vi "FPGA Main Default.vi"() -> ()   [LabVIEW 2019]
doc: "The myRIO v1.1 FPGA Shipping Personality. This personality contains support for:\n- 2 Analog Input Interrupt channel\n- 4 Digital Input Interrupt channel\n- 1 Timer\n- 1 Accelerometer\n- 1 Button\n- 4 LED\n- 10 Analog Input channels with 1 Sample\n- 6 Analog Output channels with 1 Sample\n- 40 Digital I/O channels with 1 Sample\n- 2 I2C channels\n- 4 Encoder channels\n- 6 PWM channels\n- 2 SPI channels"
uses:
  Sub VIs/Utilities/Start Boolean.ctl
  <vilib>/Platform/TimedLoop/XDataNode/timing_clust.ctl
  <vilib>/Platform/TimedLoop/XDataNode/nitl_modes.ctl
  <vilib>/Platform/TimedLoop/XDataNode/wakeup.ctl
  <vilib>/rvi/Emulation/niFpgaGetClockAttributes.vi
  <vilib>/rvi/Emulation/niFpgaSctlEmulationGetInTimedLoop.vi
  <vilib>/rvi/Emulation/niFpgaEmulationReportErrorSimple.vi
  <vilib>/rvi/eio/common/nirviEmuTemplateMethod_errors.vi
  <vilib>/rvi/Emulation/niFpgaCriticalErrorInLSC.vi
  <vilib>/rvi/Emulation/niFpgaProcessEmulError.vi
  <vilib>/rvi/Emulation/niFpgaEmulationIsFPGAContextNoSignature.vi
  <vilib>/rvi/errors/niFpgaSetErrorForExecOnDevCompSimple.vi
  <vilib>/rvi/eio/common/nirviEmuReportErrorAndStop.vi
  <vilib>/rvi/DataTransferAndStorage/Container/Common/niFpgaContainerGetUniqueNameForEmu.vi
  <vilib>/rvi/FIFO/Fifo_Resource/nirvififoEmulationSetSize.vi
  <vilib>/rvi/FIFO/Fifo_Resource/nirviFifoEmulationQueueMgr.vi
  <instcachedir>/0/nirviFifoEmulationQueueMgr_E5CAEC123FF24DC58D834DCA3CDAA9B5.lvgen/nirviFifoEmulationQueueMgr_E5CAEC123FF24DC58D834DCA3CDAA9B5_000.vi
  <vilib>/rvi/FIFO/Fifo_Resource/nirvififoEmulationDetermineInputValidOut.vi
  <vilib>/rvi/FIFO/Fifo_Resource/nirvififoEmulationCreateLock.vi
  <vilib>/rvi/FIFO/Fifo_Resource/nirvififoEmulationObtainLock.vi
  <vilib>/rvi/FIFO/Fifo_Resource/nirvififoEmulationReleaseLock.vi
  <vilib>/rvi/occurrence/nirviWaitOnOccurrenceBase.vi
  <vilib>/rvi/errors/nirviReportUnexpectedCaseInternalError.vi
  <vilib>/rvi/errors/nirviReportUnexpectedCaseInternalError (U32).vi
  <vilib>/Utility/error.llb/Clear Errors.vi
  <vilib>/rvi/DataTransferAndStorage/Container/Common/niFpgaContainerExecOnDevCompGetState.vi
  <instcachedir>/0/nirviFifoEmulationQueueMgr_E5CAEC123FF24DC58D834DCA3CDAA9B5.lvgen/nirviFifoEmulationQueueMgr_E5CAEC123FF24DC58D834DCA3CDAA9B5_001.vi
  <vilib>/rvi/interface/RandomDataEmulation/niFpgaRandomDataHandleErrors.vi
  <vilib>/rvi/DataTransferAndStorage/Container/Common/niFpgaContainerSetEmuInfo.vi
  <vilib>/eio/EIONode/EIONode.xnode
  <vilib>/rvi/DataTransferAndStorage/Container/XNode/niFpgaContainer.xnode
  <vilib>/rvi/FIFO/Fifo_Resource/nirvififoEmulationWrite.vi
  <vilib>/rvi/FIFO/Fifo_Resource/nirvififoEmulationRead.vi
  <vilib>/Platform/TimedLoop/XDataNode/XDataNode.xnode
  <vilib>/rvi/FIFO/Fifo_Resource/niFpgaFifoEmulationRefIn.vi
  <vilib>/rvi/LocalResourceManager/LocalResourceManager.xnode
  <vilib>/Platform/TimedLoop/XDataNode/XDNodeRunTimeDep.lvlib
panel:
  in  "AO.A_0.VAL":u16
  in  "AO.A_1.VAL":u16
  in  "AO.B_0.VAL":u16
  in  "AO.B_1.VAL":u16
  out "AI.B_3.VAL":u16
  out "AI.B_2.VAL":u16
  out "AI.B_1.VAL":u16
  out "AI.B_0.VAL":u16
  out "AI.A_3.VAL":u16
  out "AI.A_2.VAL":u16
  out "AI.A_1.VAL":u16
  out "AI.A_0.VAL":u16
  in  "PWM.A_2.CS":u8=1
  in  "PWM.A_2.CNFG":u8=4
  out "PWM.A_2.CNTR":u16
  in  "PWM.A_2.MAX":u16=39999
  in  "PWM.A_2.CMP":u16=20000
  in  "PWM.A_1.CS":u8=1
  in  "PWM.A_1.CNFG":u8=4
  out "PWM.A_1.CNTR":u16
  in  "PWM.A_1.MAX":u16=39999
  in  "PWM.A_1.CMP":u16=20000
  in  "PWM.A_0.CS":u8=1
  in  "PWM.A_0.CNFG":u8=4
  out "PWM.A_0.CNTR":u16
  in  "PWM.A_0.CMP":u16=20000
  in  "PWM.A_0.MAX":u16=39999
  in  "SPI.A.DATO":u16
  out "SPI.A.DATI":u16
  in  "SPI.A.CNFG":u16=112
  in  "SPI.A.CNT":u16=19
  in  "ENC.A.CNFG":u8 format="%08b"
  out "ENC.A.CNTR":u32
  out "ENC.A.STAT":u8 format="%08b"
  in  "SPI.A.GO":T1
  out "SPI.A.STAT":u8 format="%08b"
  out "I2C.A.STAT":u8 format="%08b"
  in  "I2C.A.CNTL":u8 format="%08b"
  in  "I2C.A.CNTR":u8=213
  in  "I2C.A.ADDR":u8 format="%08b"
  out "I2C.A.DATI":u8
  in  "I2C.A.DATO":u8
  in  "I2C.A.CNFG":u8=1 format="%08b"
  in  "I2C.A.GO":T1
  out "SYS.AI.RDY":bool
  out "SYS.RDY":bool
  out "DIO.A_7:0.IN":u8 format="%08b"
  in  "DIO.A_7:0.OUT":u8 format="%08b"
  in  "DIO.A_7:0.DIR":u8 format="%08b"
  out "DIO.C_7:0.IN":u8 format="%08b"
  in  "DIO.C_7:0.DIR":u8 format="%08b"
  in  "DIO.C_7:0.OUT":u8 format="%08b"
  out "AI.C_1.VAL":u16
  out "AI.C_0.VAL":u16
  in  "AO.C_0.VAL":u16
  in  "AO.C_1.VAL":u16
  in  "SYS.SELECTC":u8 format="%08b"
  in  "SYS.SELECTA":u8 format="%08b"
  in  "ENC.C_0.CNFG":u8 format="%08b"
  out "ENC.C_0.CNTR":u32
  out "ENC.C_0.STAT":u8 format="%08b"
  in  "ENC.C_1.CNFG":u8 format="%08b"
  out "ENC.C_1.CNTR":u32
  out "ENC.C_1.STAT":u8 format="%08b"
  in  "PWM.C_1.CS":u8=1
  in  "PWM.C_1.CNFG":u8=4
  out "PWM.C_1.CNTR":u16
  in  "PWM.C_1.CMP":u16=20000
  in  "PWM.C_1.MAX":u16=39999
  in  "PWM.C_0.CS":u8=1
  in  "PWM.C_0.CNFG":u8=4
  out "PWM.C_0.CNTR":u16
  in  "PWM.C_0.CMP":u16=20000
  in  "PWM.C_0.MAX":u16=39999
  out "DIO.A_15:8.IN":u8 format="%08b"
  in  "DIO.A_15:8.OUT":u8 format="%08b"
  in  "DIO.A_15:8.DIR":u8 format="%08b"
  out "AI.AudioIn_R.VAL":u16
  out "AI.AudioIn_L.VAL":u16
  in  "AO.AudioOut_R.VAL":u16
  in  "AO.AudioOut_L.VAL":u16
  in  "AO.SYS.GO":T1
  out "ACC.X.VAL":u16
  out "ACC.Y.VAL":u16
  out "SYS.ACC.RDY":bool
  out "ACC.Z.VAL":u16
  in  "DO.LED3:0":u8 format="%04b"
  out "DI.BTN":u8 format="%08b"
  out "AO.SYS.STAT":bool
  in  "IRQ.AI_A_3:0.CNFG":u8 format="%.0b"
  in  "IRQ.AI_A_0.THRESHOLD":u16
  in  "IRQ.AI_A_1.THRESHOLD":u16
  in  "IRQ.AI_A_0.NO":u8
  in  "IRQ.AI_A_1.NO":u8
  in  "IRQ.DIO_A_7:0.ENA":u8 format="%08b"
  in  "IRQ.DIO_A_7:0.RISE":u8 format="%08b"
  in  "IRQ.DIO_A_7:0.FALL":u8 format="%08b"
  in  "IRQ.DIO_A_0.NO":u8
  in  "IRQ.DIO_A_1.NO":u8
  in  "IRQ.DIO_A_2.NO":u8
  in  "IRQ.DIO_A_3.NO":u8
  in  "IRQ.DIO_A_3.CNT":u32
  in  "IRQ.DIO_A_2.CNT":u32
  in  "IRQ.DIO_A_1.CNT":u32
  in  "IRQ.DIO_A_0.CNT":u32
  in  "IRQ.AI_A_1.HYSTERESIS":u16=17
  in  "IRQ.TIMER.WRITE":u32
  in  "IRQ.TIMER.SETTIME":T1
  out "IRQ.TIMER.READ":u32
  in  "SPI.A.IRQ.NO":u8=15
  in  "IRQ.AI_A_0.HYSTERESIS":u16=17
  in  "IRQ.DI_BTN.ENA":bool
  in  "IRQ.DI_BTN.RISE":bool
  in  "IRQ.DI_BTN.FALL":bool
  in  "IRQ.DI_BTN.CNT":u32
  in  "IRQ.DI_BTN.NO":u8
  # "System"
  # "Onboard Devices"
  # "Connector A"
  # "Connector B"
  # "Connector C"
  # "Audio Connector"
  # "Accelerometer"
  # "Analog Input"
  # "Analog Output"
  # "Digital I/O"
  # "PWM"
  # "SPI Master"
  # "Analog Input"
  # "Analog Output"
  # "Digital I/O"
  # "PWM"
  # "SPI Master"
  # "Analog Input"
  # "Analog Output"
  # "Digital I/O"
  # "Counters / PWM"
  # "Analog Input"
  # "Analog Output"
  # "IO Configuration"
  # "IO Configuration"
  # "IO Configuration"
  # "Encoders"
  # "Buttons & LEDs"
  # "Analog Interrupt"
  # "Digital Interrupt"
  # "Encoders"
  # "Encoders"
  # "Button Interrupt"
  # "I2C Master"
  # "I2C Master"
  # "Timer Interrupt"
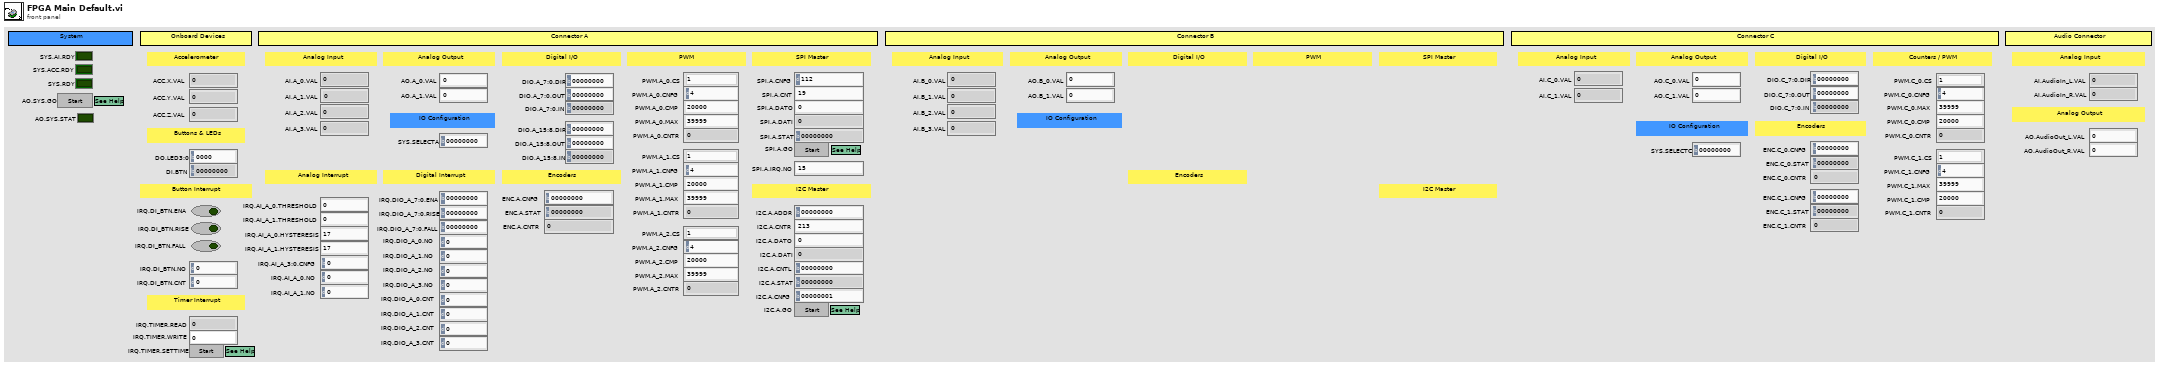
[diagram p1: front panel]
types:
  T1 = typedef "Start Boolean.ctl" = bool
  T2 = typedef "XDNodeRunTimeDep.lvlib/timing_clust.ctl" = cluster{"Expected End [f-1]":u64, "Actual End [f-1]":u64, "Finished Late? [f-1]":bool, "Expected End [i-1]":u64, "Actual End [i-1]":u64, "Finished Late? [i-1]":bool, "Expected Start [i]":u64, "Actual Start [i]":u64, "Expected Start [f]":u64, "Actual Start [f]":u64, "Source Name":string, "Structure Name":string, "Period":i64, "Deadline":i64, "Offset":i64, "Start":i64, "Priority":i32, "Timeout":i32, "Mode":T3, "Wakeup Reason":T4, "Error":errorcluster, "Source Type":string, "Secondary Source Type":string, "Global End Time":u64, "Global Start Time":u64, "Frame Duration":u64, "Iteration Duration":u64, "Assigned CPU":i32, "I/O Scan Engine Mode":u32}
  T3 = typedef "XDNodeRunTimeDep.lvlib/nitl_modes.ctl" = enum32{"No Change", "Process missed periods, maintain original phase", "Discard missed periods, maintain original phase", "Process missed periods, ignore original phase", "Discard missed periods, ignore original phase"}
  T4 = typedef "XDNodeRunTimeDep.lvlib/wakeup.ctl" = enum32{"Normal", "Aborted", "Asynchronous wakeup", "Timing source error", "Timed loop error", "Timeout"}
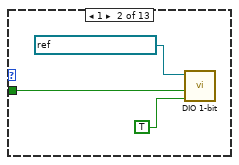
[diagram p3: hidden frame]
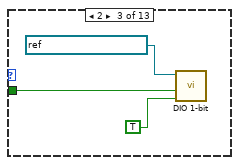
[diagram p4: hidden frame]
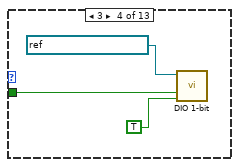
[diagram p5: hidden frame]
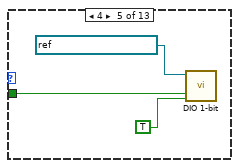
[diagram p6: hidden frame]
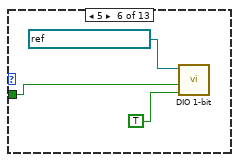
[diagram p7: hidden frame]
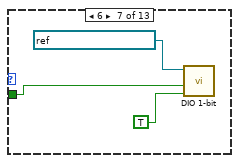
[diagram p8: hidden frame]
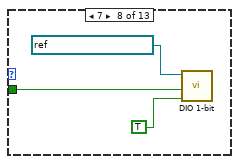
[diagram p9: hidden frame]
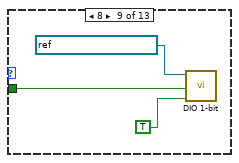
[diagram p10: hidden frame]
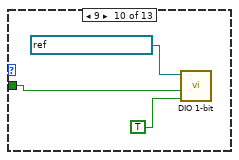
[diagram p11: hidden frame]
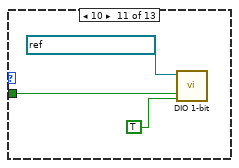
[diagram p12: hidden frame]
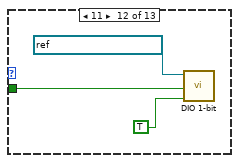
[diagram p13: hidden frame]
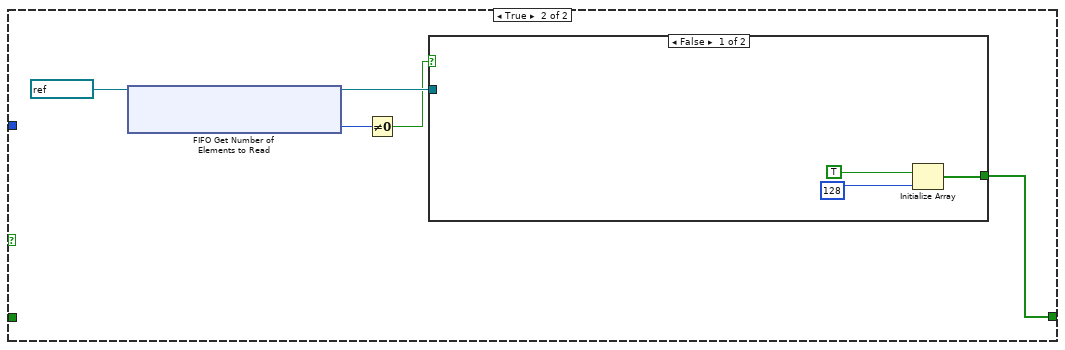
[diagram p15: hidden frame]
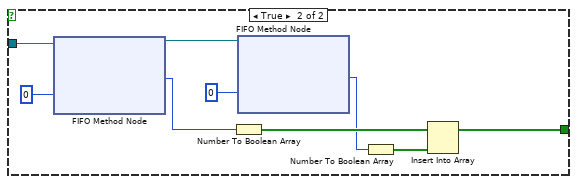
[diagram p16: hidden frame]
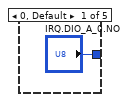
[diagram p19: hidden frame]
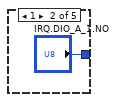
[diagram p20: hidden frame]
diagram:
  # "The Timed Loop does not allow writing the same FIFO outside the Timed Loop. Use another FIFO to push all interrupts from Button in the Timed Loop to the IRQ Queue."
  # "The Timed Loop does not allow writing the same FIFO outside the Timed Loop. Use another FIFO to push all interrupts from DIO in the Timed Loop to the IRQ Queue."
  # "The accelerometer nodes take some time before the FPGA can first read the values. This is because it takes time to read from the accelerometer. An iteration of the While Loop will not complete until the accelerometer values have been read.\n\nAfter the completion of the first iteration of the While Loop, all indicators have valid values."
  # "The analog output nodes take some time before the FPGA write the values to the pins. The GO and STAT registers are used to handshake between the FPGA and host. When the host wants the values to be written, the host sets the GO register to TRUE. If the host reads the STAT register before setting the value of the GO register, it can wait for the value of the STAT register to invert. The value inversion tells the host that the output values have been written."
  # "The analog input nodes take some time before the FPGA can first read the values. This is because it takes time to set up the Analog-to-Digital converter (ADC) and convert the first reading. An iteration of the While Loop will not complete until all the analog input channels have been sampled.\n\nAfter the completion of the first iteration of the While Loop, all indicators have valid values."
  # "Note: On some hardware a \"ghosting effect\" may occur on any unconnected AI channels. For example, if channel AI0 is connected and channels AI1~AI7 are not connected the the value read at AI0 may be seen on indicators AI1~AI7. This is common for hardware that use a multiplexed (MUXed) Analog-to-Digital converter (ADC), because the input analog signal is used to charge a capacitor which does not discharge before the unconnected channel is read.\n\nYou can hide the \"ghosting effect\" by using an mask register. This register is used to decide when the indicator should be updated."
  # "The FPGA timer fires the interrupt request (IRQ) when TIMER.Read counts down to zero. If TIMER.Read is not zero, it counts down to one per microsecond."
  # "The only interface that sends interrupts to the RT side. Timer interrupts, analog input interrupts, digital input interrupts, and SPI interrupt share this interface.\n\nAll interrupts work in sequence. One interrupt waits until the previous interrupt request (IRQ) gets acknowledged on the RT side."
  # "NOTE: The SYS.RDY Boolean MUST exist and must become TRUE at some point. Otherwise, the myRIO VIs will not function correctly."
  # "There is some delay between the time when the FPGA code starts and the time when the analog inputs, accelerometer, and scaling values outputs are valid. If the host wants to ensure that there are valid values in theses registers it should wait for each subsystem to finish its initialization process. \n\nWhen all subsystems have finished initializinig, the SYS.RDY indicator turns true. The host can poll the SYS.RDY indicator to determine the status of the FPGA. Alternatively, the host can poll the individual SYS.xx.RDY indicators to determine the status of the individual subsystems.\n\nThis loop continues indefinitely, essentially making SYS.RDY a read-only register."
  n1 = while {
    stop <- FALSE stop-if-true
    # "Host Synchronization"
    n2 = local read "SYS.ACC.RDY"() -> (w13:bool)
    n3 = local read "SYS.AI.RDY"() -> (w15:bool)
    n4 = Compound Arithmetic op=AND(w15, w13) -> (→"SYS.RDY":bool)
  }
  n5 = while {
    stop <- FALSE stop-if-true
    # "Interrupt to RT"
    n6 = xnode ("FIFO Method Node")("Timeout"=-1) -> ("Element"=w18:u8)  [unwired: 1 in, 2 out]
    n7 = call <vilib>:"niFPGA Interrupt.vi"("Wait Until Cleared (F)"=TRUE, "IRQ Number (0)"=w18) -> ()  [unwired: 1 in]
  }
  n8 = while {
    stop <- FALSE stop-if-true
    # "Timer"
    n9 = local read "IRQ.TIMER.READ"() -> (w23:u32)
    n10 = Select(t="IRQ.TIMER.WRITE", s="IRQ.TIMER.SETTIME", f=w23) -> (s? t:f=w21:u32)
    n11 = case shown="Default" w21 {
      selector: w21 -> [w27 w30]
      tunnel: [w27 w28] -> w20
      frame 0 {
      }
      frame Default {
        n12 = Decrement(x=w30) -> (x-1=w29:u32)
        n13 = case shown="0" w29 {
          selector: w29 -> [w31 w34]
          tunnel: [w31 w34] -> w28
          frame Default {
          }
          frame 0 {
            w33 = u8 0  # Reserved for Timer IRQ
            n14 = xnode ("FIFO Method Node")("Element"=w33, "Timeout"=-1) -> ()  [unwired: 1 in, 2 out]
          }
        }
      }
    }
    "IRQ.TIMER.READ" <- w20
    n15 = call "Loop Timer"("Count(uSec)"=u8 1 ("Count(mSec)")) -> ()  [unwired: 1 out]
  }
  n16 = xnode "VI-Defined FIFO Configuration"() -> ("FIFO Out"=w3:refnum<k21>)
  n17 = while {
    tunnel: w3 -> [w36]
    i -> [w63]
    stop <- FALSE stop-if-true
    # "Analog Input"
    n18 = xnode "FPGA I/O Node"() -> ("ConnectorA/AI0"=w41:u16, "ConnectorA/AI1"=w40:u16, "ConnectorA/AI2"=→"AI.A_2.VAL":u16, "ConnectorA/AI3"=→"AI.A_3.VAL":u16, "ConnectorB/AI0"=→"AI.B_0.VAL":u16, "ConnectorB/AI1"=→"AI.B_1.VAL":u16, "ConnectorB/AI2"=→"AI.B_2.VAL":u16, "ConnectorB/AI3"=→"AI.B_3.VAL":u16, "ConnectorC/AI0"=w57:i16, "ConnectorC/AI1"=w56:i16, "AudioIn/Left"=w55:i16, "AudioIn/Right"=w54:i16)  [unwired: 12 in, 12 out]
    "AI.A_0.VAL" <- w41
    "AI.A_1.VAL" <- w40
    n19 = Greater Than 0?(x=w63) -> (x > 0?=→"SYS.AI.RDY":bool)
    n20 = Number To Boolean Array(number="IRQ.AI_A_3:0.CNFG") -> (Boolean array=w51:bool[])
    n21 = Index Array(array=w51) -> (element #1=w49:bool, element #2=w48:bool, element #3=w46:bool, element #4=w45:bool)  [unwired: 4 in]
    n22 = To Unsigned Word Integer(number=w57) -> (unsigned 16bit integer=→"AI.C_0.VAL":u16)
    n23 = To Unsigned Word Integer(number=w56) -> (unsigned 16bit integer=→"AI.C_1.VAL":u16)
    n24 = To Unsigned Word Integer(number=w55) -> (unsigned 16bit integer=→"AI.AudioIn_L.VAL":u16)
    n25 = To Unsigned Word Integer(number=w54) -> (unsigned 16bit integer=→"AI.AudioIn_R.VAL":u16)
    n26 = call "Check AI IRQ.vi"("Hysteresis"="IRQ.AI_A_1.HYSTERESIS", "FIFO In"=w36, "IRQ Number"="IRQ.AI_A_1.NO", "Threshold"="IRQ.AI_A_1.THRESHOLD", "Analog Value"=w40, "Rising Edge?"=w45, "Enable Interrupt?"=w46) -> ()  [unwired: 5 in]
    n27 = call "Check AI IRQ.vi"("Hysteresis"="IRQ.AI_A_0.HYSTERESIS", "FIFO In"=w36, "IRQ Number"="IRQ.AI_A_0.NO", "Threshold"="IRQ.AI_A_0.THRESHOLD", "Analog Value"=w41, "Rising Edge?"=w48, "Enable Interrupt?"=w49) -> ()  [unwired: 5 in]
  }
  n28 = while {
    stop <- FALSE stop-if-true
    # "Analog Output"
    n29 = feedback #1(FALSE) -> (w69:bool)
    n30 = case shown="True" "AO.SYS.GO" {
      tunnel: "AO.C_0.VAL" -> [_ w91]
      tunnel: "AO.C_1.VAL" -> [_ w90]
      tunnel: "AO.A_0.VAL" -> [_ w95]
      tunnel: "AO.A_1.VAL" -> [_ w94]
      tunnel: "AO.B_0.VAL" -> [_ w93]
      tunnel: "AO.B_1.VAL" -> [_ w92]
      tunnel: "AO.AudioOut_L.VAL" -> [_ w87]
      tunnel: "AO.AudioOut_R.VAL" -> [_ w86]
      tunnel: w69 -> [w80 w83]
      tunnel: [w80 w81] -> w67
      frame False {
      }
      frame True {
        n31 = To Word Integer(number=w91) -> (16bit integer=w89:i16)
        n32 = To Word Integer(number=w90) -> (16bit integer=w88:i16)
        n33 = To Word Integer(number=w87) -> (16bit integer=w85:i16)
        n34 = To Word Integer(number=w86) -> (16bit integer=w84:i16)
        n35 = flat-sequence {
          tunnel: w95 -> [w104]
          tunnel: w94 -> [w103]
          tunnel: w93 -> [w102]
          tunnel: w92 -> [w101]
          tunnel: w89 -> [w100]
          tunnel: w88 -> [w99]
          tunnel: w85 -> [w98]
          tunnel: w84 -> [w97]
          tunnel: w83 -> [w96]
          tunnel: [w96] -> w82
          tunnel: w82 -> [w106]
          tunnel: [w105] -> w81
          frame #0 {
            n36 = xnode "FPGA I/O Node"("ConnectorA/AO0"=w104, "ConnectorA/AO1"=w103, "ConnectorB/AO0"=w102, "ConnectorB/AO1"=w101, "ConnectorC/AO0"=w100, "ConnectorC/AO1"=w99, "AudioOut/Left"=w98, "AudioOut/Right"=w97) -> ()  [unwired: 8 in, 8 out]
          }
          frame #1 {
            n37 = Not(x=w106) -> (.not. x?=w105:bool)
          }
        }
      }
    }
    "AO.SYS.STAT" <- w67
    n38 = feedback-in #1(w67) -> ()
  }
  n39 = while {
    i -> [w111]
    stop <- FALSE stop-if-true
    # "Onboard Accelerometer"
    n40 = xnode "FPGA I/O Node"() -> ("AccelerationX"=w114:i16, "AccelerationY"=w113:i16, "AccelerationZ"=w112:i16)  [unwired: 3 in, 3 out]
    n41 = Greater Than 0?(x=w111) -> (x > 0?=→"SYS.ACC.RDY":bool)
    n42 = To Unsigned Word Integer(number=w114) -> (unsigned 16bit integer=→"ACC.X.VAL":u16)
    n43 = To Unsigned Word Integer(number=w113) -> (unsigned 16bit integer=→"ACC.Y.VAL":u16)
    n44 = To Unsigned Word Integer(number=w112) -> (unsigned 16bit integer=→"ACC.Z.VAL":u16)
  }
  n45 = xnode "VI-Defined FIFO Configuration"() -> ("FIFO Out"=w2:refnum<k21>)
  n46 = node-c288() -> (w5:T2)  [unwired: 1 in]
  n47 = timed-loop {
    timing: w5 -> [_]
    timing-out: [_] -> w4
    tunnel: w2 -> [w118]
    stop <- _ stop-if-true
    # "Onboard DIO"
    n48 = xnode "FPGA I/O Node"() -> ("Button0"=w122:bool)  [unwired: 1 in, 1 out]
    n49 = Number To Boolean Array(number="DO.LED3:0") -> (Boolean array=w127:bool[])
    n50 = Build Array(w122) -> (w130:bool[])
    n51 = Index Array(array=w127) -> (element #1=w126:bool, element #2=w125:bool, element #3=w124:bool, element #4=w123:bool)  [unwired: 4 in]
    n52 = call "DIO IRQ 1-bit.vi"("IRQ.NO"="IRQ.DI_BTN.NO", "IRQ.CNT"="IRQ.DI_BTN.CNT", "FIFO in"=w118, "IRQ.FALL"="IRQ.DI_BTN.FALL", "IRQ.RISE"="IRQ.DI_BTN.RISE", "IRQ.ENA"="IRQ.DI_BTN.ENA", "DIO"=w122) -> ()  [unwired: 5 in]
    n53 = Boolean Array To Number(Boolean array=w130) -> (number=→"DI.BTN":u8)
    n54 = xnode "FPGA I/O Node"("LED0"=w126, "LED1"=w125, "LED2"=w124, "LED3"=w123) -> ()  [unwired: 4 in, 4 out]
  }
  n55 = while {
    stop <- FALSE stop-if-true
    # "Button SCTL Interrupt Buffer"
    n56 = feedback #2(u8 0 ("Element")) -> (w135:u8)
    n57 = feedback #3(FALSE ("Timed Out?")) -> (w139:bool)
    n58 = case shown="False" w139 {
      tunnel: [w141 w143] -> w136
      tunnel: w135 -> [_ w143]
      frame False {
        n59 = xnode ("FIFO Method Node")("Timeout"=-1) -> ("Element"=w141:u8)  [unwired: 1 in, 2 out]
      }
      frame True {
      }
    }
    n60 = feedback-in #2(w136) -> ()
    n61 = xnode ("FIFO Method Node")("Element"=w136, "Timeout"=0) -> ("Timed Out?"=w137:bool)  [unwired: 1 in, 1 out]
    n62 = feedback-in #3(w137) -> ()
  }
  n63 = node-c288(w4) -> ()
  n64 = xnode "VI-Defined FIFO Configuration"() -> ()  [unwired: 1 out]
  n65 = node-c288() -> (w9:T2)  [unwired: 1 in]
  n66 = timed-loop {
    timing: w9 -> [_]
    timing-out: [_] -> w8
    stop <- _ stop-if-true
    w144 = u16 5 ("Debounce Ticks")
    w145 = u8 0
    # "Trigger the interrupt at next \ntick if timeout"
    # "DIO / Encoder"
    # "DIO / I2C Master"
    # "DIO / PWM"
    # "DIO"
    # "DIO"
    # "DIO/ SPI Master"
    # "Connector A DIO"
    n67 = call "Split HDC Bank1 DIO.vi"("IN 7:0"="DIO.A_7:0.OUT") -> ("OUT 3:0"=w280:fxp<+,4,4>, "OUT 4"=w199:bool, "OUT 7:5"=w277:fxp<+,3,3>)
    n68 = call "Split HDC Bank1 DIO.vi"("IN 7:0"="DIO.A_7:0.DIR") -> ("OUT 3:0"=w279:fxp<+,4,4>, "OUT 4"=w278:bool, "OUT 7:5"=w276:fxp<+,3,3>)
    n69 = call "Split HDC Function Select.vi"("IN 7:0"="SYS.SELECTA") -> ("OUT 1:0"=w219:fxp<+,2,2>, "OUT 7"=w214:bool, "OUT 2"=w218:bool, "OUT 3"=w217:bool, "OUT 4"=w216:bool, "OUT 5"=w215:bool)
    n70 = call "DIO 4-bit.vi"("DIO0 Refnum"=refnum<k21> "ConnectorA/DIO0", "DIO1 Refnum"=refnum<k21> "ConnectorA/DIO1", "DIO2 Refnum"=refnum<k21> "ConnectorA/DIO2", "DIR 3:0"=w279, "OUT 3:0"=w280, "DIO3 Refnum"=refnum<k21> "ConnectorA/DIO3") -> ("IN 3:0"=w167:fxp<+,4,4>)  [unwired: 5 in]
    n71 = call "DIO 1-bit.vi"("DIR"=w278, "OUT"=w199, "DIO Refnum"=refnum<k21> "ConnectorA/DIO4") -> ("IN"=w166:bool)  [unwired: 8 in]
    n72 = call "DIO_SPI.vi"("DIO.2:0.OUT"=w277, "DIO.2:0.DIR"=w276, "SPI.CNT"="SPI.A.CNT", "SPI.CNFG"="SPI.A.CNFG", "SPI.DATO"="SPI.A.DATO", "SPI.GO"="SPI.A.GO", "DIO.2/SPI.MOSI Refnum"=refnum<k21> "ConnectorA/DIO7" ("DIO.2/SPI.SCLK"), "SELECT.1:0"=w219, "DIO.1/SPI.MISO Refnum"=refnum<k21> "ConnectorA/DIO6" ("DIO.1/SPI.MOSI"), "DIO.0/SPI.SCLK Refnum"=refnum<k21> "ConnectorA/DIO5" ("DIO.0/SPI.MISO")) -> ("DIO.2:0.IN"=w252:fxp<+,3,3>, "SPI.DATI"=→"SPI.A.DATI":u16, "SPI.STAT"=w152:u8)  [unwired: 7 in]
    "SPI.A.STAT" <- w152
    n73 = Number To Boolean Array(number=w152) -> (Boolean array=w154:bool[])
    n74 = Index Array(array=w154) -> (element=w153:bool)  [unwired: 1 in]
    n75 = call "Falling Edge Trigger.vi"("Signal"=w153) -> ("Trigger?"=w151:bool)
    n76 = call "Join HDC Bank1 DIO.vi"("IN 7:5"=w252, "IN 4"=w166, "IN 3:0"=w167) -> ("OUT 7:0"=→"DIO.A_7:0.IN":u8)
    n77 = Number To Boolean Array(number=w167) -> (Boolean array=w192:bool[])
    n78 = Number To Boolean Array(number="IRQ.DIO_A_7:0.ENA") -> (Boolean array=w198:bool[])
    n79 = Number To Boolean Array(number="IRQ.DIO_A_7:0.RISE") -> (Boolean array=w197:bool[])
    n80 = Number To Boolean Array(number="IRQ.DIO_A_7:0.FALL") -> (Boolean array=w196:bool[])
    n81 = call "Split HDC Bank2 DIO.vi"("IN 7:0"="DIO.A_15:8.OUT") -> ("OUT 5"=w201:bool, "OUT 7:6"=w223:fxp<+,2,2>, "OUT 4:3"=w203:fxp<+,2,2>, "OUT 2"=w205:bool, "OUT 0"=w209:bool, "OUT 1"=w208:bool)  [unwired: 2 in]
    n82 = call "Split HDC Bank2 DIO.vi"("IN 7:0"="DIO.A_15:8.DIR") -> ("OUT 5"=w200:bool, "OUT 7:6"=w222:fxp<+,2,2>, "OUT 4:3"=w202:fxp<+,2,2>, "OUT 2"=w204:bool, "OUT 0"=w207:bool, "OUT 1"=w206:bool)  [unwired: 2 in]
    n83 = Index Array(array=w192) -> (element #1=w173:bool, element #2=w188:bool, element #3=w187:bool, element #4=w186:bool)  [unwired: 4 in]
    n84 = Index Array(array=w198) -> (element #1=w191:bool, element #2=w185:bool, element #3=w184:bool, element #4=w183:bool)  [unwired: 4 in]
    n85 = Index Array(array=w197) -> (element #1=w190:bool, element #2=w182:bool, element #3=w181:bool, element #4=w180:bool)  [unwired: 4 in]
    n86 = Index Array(array=w196) -> (element #1=w189:bool, element #2=w179:bool, element #3=w178:bool, element #4=w177:bool)  [unwired: 4 in]
    n87 = call "Check DI IRQ.vi"("Debounce Ticks"=w144, "Count"="IRQ.DIO_A_0.CNT", "On Falling Edge?"=w189, "On Rising Edge?"=w190, "Enable Interrupt?"=w191, "Digital In"=w173) -> ("Trigger?"=w164:bool)  [unwired: 5 in]
    n88 = call "Check DI IRQ.vi"("Debounce Ticks"=w144, "Count"="IRQ.DIO_A_1.CNT", "On Falling Edge?"=w179, "On Rising Edge?"=w182, "Enable Interrupt?"=w185, "Digital In"=w188) -> ("Trigger?"=w163:bool)  [unwired: 5 in]
    n89 = call "Check DI IRQ.vi"("Debounce Ticks"=w144, "Count"="IRQ.DIO_A_2.CNT", "On Falling Edge?"=w178, "On Rising Edge?"=w181, "Enable Interrupt?"=w184, "Digital In"=w187) -> ("Trigger?"=w162:bool)  [unwired: 5 in]
    n90 = call "DIO_PWM.vi"("DIO.OUT"=w209, "DIO.DIR"=w207, "PWM.CS"="PWM.A_0.CS", "PWM.CNFG"="PWM.A_0.CNFG", "PWM.CMP"="PWM.A_0.CMP", "PWM.MAX"="PWM.A_0.MAX", "DIO/PWM"=refnum<k21> "ConnectorA/DIO8", "SELECT"=w218) -> ("DIO.IN"=w213:bool, "PWM.CNTR"=→"PWM.A_0.CNTR":u16)  [unwired: 10 in]
    n91 = call "DIO_PWM.vi"("DIO.OUT"=w208, "DIO.DIR"=w206, "PWM.CS"="PWM.A_1.CS", "PWM.CNFG"="PWM.A_1.CNFG", "PWM.CMP"="PWM.A_1.CMP", "PWM.MAX"="PWM.A_1.MAX", "DIO/PWM"=refnum<k21> "ConnectorA/DIO9", "SELECT"=w217) -> ("DIO.IN"=w212:bool, "PWM.CNTR"=→"PWM.A_1.CNTR":u16)  [unwired: 10 in]
    n92 = call "DIO_PWM.vi"("DIO.OUT"=w205, "DIO.DIR"=w204, "PWM.CS"="PWM.A_2.CS", "PWM.CNFG"="PWM.A_2.CNFG", "PWM.CMP"="PWM.A_2.CMP", "PWM.MAX"="PWM.A_2.MAX", "DIO/PWM"=refnum<k21> "ConnectorA/DIO10", "SELECT"=w216) -> ("DIO.IN"=w211:bool, "PWM.CNTR"=→"PWM.A_2.CNTR":u16)  [unwired: 10 in]
    n93 = call "Check DI IRQ.vi"("Debounce Ticks"=w144, "Count"="IRQ.DIO_A_3.CNT", "On Falling Edge?"=w177, "On Rising Edge?"=w180, "Enable Interrupt?"=w183, "Digital In"=w186) -> ("Trigger?"=w161:bool)  [unwired: 5 in]
    n94 = feedback #4(w145) -> (w147:u8)
    n95 = Less?(x=w147, y=4 ("x")) -> (x < y?=w149:bool)
    n96 = Increment(x=w147) -> (x+1=w148:u8)
    n97 = Select(t=w148, s=w149, f=w145) -> (s? t:f=w146:u8)
    n98 = feedback-in #4(w146) -> ()
    n99 = case shown="4" w147 {
      tunnel: ["IRQ.DIO_A_0.NO" "IRQ.DIO_A_1.NO" "IRQ.DIO_A_2.NO" "IRQ.DIO_A_3.NO" "SPI.A.IRQ.NO"] -> w176
      frame 0, Default {
      }
      frame 1 {
      }
      frame 2 {
      }
      frame 3 {
      }
      frame 4 {
      }
    }
    n100 = Build Array(w164, w163, w162, w161, w151) -> (w159:bool[])
    n101 = call "DIO_Encoder.vi"("DIO.1:0.OUT"=w203, "DIO.1:0.DIR"=w202, "QE.CNFG"="ENC.A.CNFG", "DIO.1/QE.B"=refnum<k21> "ConnectorA/DIO12", "SELECT"=w215, "DIO.0/QE.A"=refnum<k21> "ConnectorA/DIO11") -> ("DIO.1:0.IN"=w210:fxp<+,2,2>, "QE.CNTR"=→"ENC.A.CNTR":u32, "QE.STAT"=→"ENC.A.STAT":u8)  [unwired: 11 in]
    n102 = call "DIO 1-bit.vi"("DIR"=w200, "OUT"=w201, "DIO Refnum"=refnum<k21> "ConnectorA/DIO13") -> ("IN"=w165:bool)  [unwired: 8 in]
    n103 = call "DIO_I2C.vi"("DIO.1:0.OUT"=w223, "DIO.1:0.DIR"=w222, "I2C.CNFG"="I2C.A.CNFG", "I2C.CNTL"="I2C.A.CNTL", "I2C.ADDR"="I2C.A.ADDR", "I2C.DATO"="I2C.A.DATO", "DIO.1/I2C.SDA"=refnum<k21> "ConnectorA/DIO15" ("DIO.1/I2C.SCL"), "I2C.CNTR"="I2C.A.CNTR", "DIO.0/I2C.SCL"=refnum<k21> "ConnectorA/DIO14" ("DIO.0/I2C.SDA"), "Execute?"="I2C.A.GO", "SELECT"=w214) -> ("DIO.1:0.IN"=w221:fxp<+,2,2>, "I2C.DATI"=→"I2C.A.DATI":u8, "I2C.STAT"=→"I2C.A.STAT":u8)  [unwired: 6 in]
    n104 = feedback #5(bool[] [FALSE, FALSE, FALSE, FALSE, FALSE] ("initialized array")) -> (w155:bool[])
    n105 = Or(x=w159, y=w155) -> (x .or. y?=w160:bool[])
    n106 = Index Array(array=w160, index=w147) -> (element=w158:bool)
    n107 = case shown="True" w158 {
      selector: w158 -> [w281 _]
      tunnel: [w281 w282] -> w157
      tunnel: w176 -> [_ w283]
      frame False {
      }
      frame True {
        n108 = xnode ("FIFO Method Node")("Element"=w283, "Timeout"=0) -> ("Timed Out?"=w282:bool)  [unwired: 1 in, 1 out]
      }
    }
    n109 = Replace Array Subset(array=w160, new element=w157, index=w147) -> (w156:bool[])
    n110 = feedback-in #5(w156) -> ()
    n111 = call "Join HDC Bank2 DIO.vi"("IN 7:6"=w221, "IN 5"=w165, "IN 4:3"=w210, "IN 0"=w213, "IN 2"=w211, "IN 1"=w212) -> ("OUT 7:0"=→"DIO.A_15:8.IN":u8)  [unwired: 4 in]
  }
  n112 = while {
    stop <- FALSE stop-if-true
    # "Connector A SCTL Interrupt Buffer"
    n113 = feedback #6(u8 0 ("Element")) -> (w294:u8)
    n114 = feedback #7(FALSE ("Timed Out?")) -> (w298:bool)
    n115 = case shown="False" w298 {
      tunnel: [w300 w302] -> w295
      tunnel: w294 -> [_ w302]
      frame False {
        n116 = xnode ("FIFO Method Node")("Timeout"=-1) -> ("Element"=w300:u8)  [unwired: 1 in, 2 out]
      }
      frame True {
      }
    }
    n117 = feedback-in #6(w295) -> ()
    n118 = xnode ("FIFO Method Node")("Element"=w295, "Timeout"=0) -> ("Timed Out?"=w296:bool)  [unwired: 1 in, 1 out]
    n119 = feedback-in #7(w296) -> ()
  }
  n120 = node-c288(w8) -> ()
  n121 = node-c288() -> (w7:T2)  [unwired: 1 in]
  n122 = timed-loop {
    timing: w7 -> [_]
    timing-out: [_] -> w6
    shift-right: [w310] -> _
    shift-left: i16 -1 -> [w307]
    stop <- _ stop-if-true
    # "Connector B DIO"
    n123 = Add(x=w307, y=i16 1) -> (x+y=w309:i16)
    n124 = Equal?(x=w309, y=i16 399) -> (x = y?=w303:bool)
    n125 = Equal To 0?(x=w309) -> (x = 0?=w305:bool)
    n126 = case shown="True" w303 {
      tunnel: [w390 i16 -1] -> w310
      tunnel: w309 -> [w390 _]
      frame False {
      }
      frame True {
      }
    }
    n127 = Initialize Array(TRUE, i16 128) -> (w311:bool[])
    n128 = feedback #8(w311) -> (w312:bool[])
    n129 = case shown="False" w305 {
      tunnel: w309 -> [w322 _]
      tunnel: w312 -> [w317 _]
      tunnel: [w317 w373] -> w304
      frame False {
        n130 = Quotient & Remainder(x=w322, y=40 ("length")) -> (x-y*floor(x/y)=w316:i32, floor(x/y)=w321:i32)
        n131 = Not Equal To 0?(x=w316) -> (x != 0?=w320:bool)
        n132 = Less Or Equal?(x=w316, y=i16 12) -> (x <= y?=w319:bool)
        n133 = And(x=w320, y=w319) -> (x .and. y?=w318:bool)
        n134 = case shown="True" w318 {
          tunnel: w316 -> [_ w332]
          tunnel: w317 -> [_ w328]
          tunnel: w321 -> [_ w327]
          frame False {
          }
          frame True {
            # "stop bit"
            # "start bit"
            n135 = Subtract(x=w332, y=1 ("length")) -> (x-y=w325:i32)
            n136 = Multiply(x=w325, y=8 ("length")) -> (x*y=w329:i32)
            n137 = Array Subset(array=w328, index=w329, length=8) -> (w334:bool[])
            n138 = Build Array (concatenate)(FALSE, w334, TRUE ("element")) -> (w326:bool[])
            n139 = Index Array(array=w326, index=w327) -> (element=w324:bool)
            n140 = case shown="0" w325 {
              tunnel: w324 -> [w337 w340 w343 w346 w349 w352 w355 w358 w361 w364 w367 w370 _]
              frame 0 {
                n141 = call "DIO 1-bit.vi"("DIR"=TRUE, "OUT"=w337, "DIO Refnum"=refnum<k21> "ConnectorB/DIO0") -> ()  [unwired: 8 in, 1 out]
              }
              frame 1 {
                n142 = call "DIO 1-bit.vi"("DIR"=TRUE, "OUT"=w340, "DIO Refnum"=refnum<k21> "ConnectorB/DIO1") -> ()  [unwired: 8 in, 1 out]
              }
              frame 2 {
                n143 = call "DIO 1-bit.vi"("DIR"=TRUE, "OUT"=w343, "DIO Refnum"=refnum<k21> "ConnectorB/DIO2") -> ()  [unwired: 8 in, 1 out]
              }
              frame 3 {
                n144 = call "DIO 1-bit.vi"("DIR"=TRUE, "OUT"=w346, "DIO Refnum"=refnum<k21> "ConnectorB/DIO3") -> ()  [unwired: 8 in, 1 out]
              }
              frame 4 {
                n145 = call "DIO 1-bit.vi"("DIR"=TRUE, "OUT"=w349, "DIO Refnum"=refnum<k21> "ConnectorB/DIO4") -> ()  [unwired: 8 in, 1 out]
              }
              frame 5 {
                n146 = call "DIO 1-bit.vi"("DIR"=TRUE, "OUT"=w352, "DIO Refnum"=refnum<k21> "ConnectorB/DIO5") -> ()  [unwired: 8 in, 1 out]
              }
              frame 6 {
                n147 = call "DIO 1-bit.vi"("DIR"=TRUE, "OUT"=w355, "DIO Refnum"=refnum<k21> "ConnectorB/DIO6") -> ()  [unwired: 8 in, 1 out]
              }
              frame 7 {
                n148 = call "DIO 1-bit.vi"("DIR"=TRUE, "OUT"=w358, "DIO Refnum"=refnum<k21> "ConnectorB/DIO7") -> ()  [unwired: 8 in, 1 out]
              }
              frame 8 {
                n149 = call "DIO 1-bit.vi"("DIR"=TRUE, "OUT"=w361, "DIO Refnum"=refnum<k21> "ConnectorB/DIO8") -> ()  [unwired: 8 in, 1 out]
              }
              frame 9 {
                n150 = call "DIO 1-bit.vi"("DIR"=TRUE, "OUT"=w364, "DIO Refnum"=refnum<k21> "ConnectorB/DIO9") -> ()  [unwired: 8 in, 1 out]
              }
              frame 10 {
                n151 = call "DIO 1-bit.vi"("DIR"=TRUE, "OUT"=w367, "DIO Refnum"=refnum<k21> "ConnectorA/DIO10") -> ()  [unwired: 8 in, 1 out]
              }
              frame 11 {
                n152 = call "DIO 1-bit.vi"("DIR"=TRUE, "OUT"=w370, "DIO Refnum"=refnum<k21> "ConnectorA/DIO11") -> ()  [unwired: 8 in, 1 out]
              }
              frame Default {
              }
            }
          }
        }
      }
      frame True {
        n153 = xnode ("FIFO Get Number of Elements to Read")("FIFO In"=refnum<k21> "UART0") -> ("Number of Elements to Read"=w376:u32, "FIFO Out"=w375:refnum<k21>)
        n154 = Not Equal To 0?(x=w376) -> (x != 0?=w374:bool)
        n155 = case shown="False" w374 {
          tunnel: w375 -> [_ w389]
          tunnel: [w378 w381] -> w373
          frame False {
            n156 = Initialize Array(TRUE, i16 128) -> (w378:bool[])
          }
          frame True {
            n157 = xnode ("FIFO Method Node")("Timeout"=0, "FIFO In"=w389) -> ("Element"=w385:u64, "FIFO Out"=w387:refnum<k21>)  [unwired: 1 out]
            n158 = Number To Boolean Array(number=w385) -> (Boolean array=w384:bool[])
            n159 = xnode ("FIFO Method Node")("Timeout"=0, "FIFO In"=w387) -> ("Element"=w383:u64)  [unwired: 2 out]
            n160 = Number To Boolean Array(number=w383) -> (Boolean array=w382:bool[])
            n161 = Insert Into Array(array=w384, new element=w382) -> (w381:bool[])  [unwired: 1 in]
          }
        }
      }
    }
    n162 = feedback-in #8(w304) -> ()
  }
  n163 = node-c288(w6) -> ()
  n164 = node-c288() -> (w11:T2)  [unwired: 1 in]
  n165 = timed-loop {
    timing: w11 -> [_]
    timing-out: [_] -> w10
    stop <- _ stop-if-true
    # "Connector C  DIO"
    n166 = call "Split myDAQ DIO.vi"("IN 7:0"="DIO.C_7:0.OUT") -> ("OUT 2, OUT0"=w412:fxp<+,2,2>, "OUT 1"=w411:bool, "OUT 3"=w410:bool, "OUT 7"=w407:bool, "OUT 6, OUT 4"=w409:fxp<+,2,2>, "OUT 5"=w408:bool)  [unwired: 4 in]
    n167 = call "Split myDAQ DIO.vi"("IN 7:0"="DIO.C_7:0.DIR") -> ("OUT 2, OUT0"=w406:fxp<+,2,2>, "OUT 1"=w405:bool, "OUT 3"=w404:bool, "OUT 7"=w401:bool, "OUT 6, OUT 4"=w403:fxp<+,2,2>, "OUT 5"=w402:bool)  [unwired: 4 in]
    n168 = call "Split myDAQ Function Select.vi"("IN 7:0"="SYS.SELECTC") -> ("OUT 0"=w418:bool, "OUT 1"=w417:bool, "OUT 2"=w416:bool, "OUT 3"=w415:bool)  [unwired: 2 in]
    n169 = call "DIO_Encoder.vi"("DIO.1:0.OUT"=w412, "DIO.1:0.DIR"=w406, "QE.CNFG"="ENC.C_0.CNFG", "DIO.1/QE.B"=refnum<k21> "ConnectorC/DIO2", "SELECT"=w418, "DIO.0/QE.A"=refnum<k21> "ConnectorC/DIO0") -> ("DIO.1:0.IN"=w399:fxp<+,2,2>, "QE.CNTR"=→"ENC.C_0.CNTR":u32, "QE.STAT"=→"ENC.C_0.STAT":u8)  [unwired: 11 in]
    n170 = call "DIO 1-bit.vi"("DIR"=w405, "OUT"=w411, "DIO Refnum"=refnum<k21> "ConnectorC/DIO1") -> ("IN"=w398:bool)  [unwired: 8 in]
    n171 = call "DIO_PWM.vi"("DIO.OUT"=w410, "DIO.DIR"=w404, "PWM.CS"="PWM.C_0.CS", "PWM.CNFG"="PWM.C_0.CNFG", "PWM.CMP"="PWM.C_0.CMP", "PWM.MAX"="PWM.C_0.MAX", "DIO/PWM"=refnum<k21> "ConnectorC/DIO3", "SELECT"=w417) -> ("DIO.IN"=w397:bool, "PWM.CNTR"=→"PWM.C_0.CNTR":u16)  [unwired: 10 in]
    n172 = call "DIO_Encoder.vi"("DIO.1:0.OUT"=w409, "DIO.1:0.DIR"=w403, "QE.CNFG"="ENC.C_1.CNFG", "DIO.1/QE.B"=refnum<k21> "ConnectorC/DIO6", "SELECT"=w416, "DIO.0/QE.A"=refnum<k21> "ConnectorC/DIO4") -> ("DIO.1:0.IN"=w396:fxp<+,2,2>, "QE.CNTR"=→"ENC.C_1.CNTR":u32, "QE.STAT"=→"ENC.C_1.STAT":u8)  [unwired: 11 in]
    n173 = call "DIO 1-bit.vi"("DIR"=w402, "OUT"=w408, "DIO Refnum"=refnum<k21> "ConnectorC/DIO5") -> ("IN"=w395:bool)  [unwired: 8 in]
    n174 = call "DIO_PWM.vi"("DIO.OUT"=w407, "DIO.DIR"=w401, "PWM.CS"="PWM.C_1.CS", "PWM.CNFG"="PWM.C_1.CNFG", "PWM.CMP"="PWM.C_1.CMP", "PWM.MAX"="PWM.C_1.MAX", "DIO/PWM"=refnum<k21> "ConnectorC/DIO7", "SELECT"=w415) -> ("DIO.IN"=w394:bool, "PWM.CNTR"=→"PWM.C_1.CNTR":u16)  [unwired: 10 in]
    n175 = call "Join myDAQ DIO.vi"("IN 7"=w394, "IN 5"=w395, "IN 6, IN 4"=w396, "IN 2, IN 0"=w399, "IN 3"=w397, "IN 1"=w398) -> ("IN 7:0"=→"DIO.C_7:0.IN":u8)  [unwired: 4 in]
  }
  n176 = node-c288(w10) -> ()
